vi "Create Runtime Configuration Files.vi"(6 "File Path":path=path "C:/dev/niveristand-runtime-configuration-example/Examples/Assets/Runtime Configuration - Subset.nivsruntimeconfig", 7 "Version":string="1.0", 8 "Error in":errorcluster, 9 "Creator":string="National Instruments", 10 "Description":string="Contains a sub set of channel information of Runtime Configuration Demo Custom Device which can be imported at runtime.", 11 "Name":string="TestRuntimeConfig") -> (0 "Error out":errorcluster)   [LabVIEW 2026]
uses:
  <vilib>/NI VeriStand/Custom Device API/Custom Device Channel Type.ctl
  <vilib>/NI/NI VeriStand Runtime Configuration File API/Runtime Configuration File API.lvlib
  <vilib>/NI VeriStand/Custom Device API/Custom Device API.lvlib
  Source/Runtime Configuration Support Example/Scripting/NIVS Runtime Configuration File Scripting API.lvlib
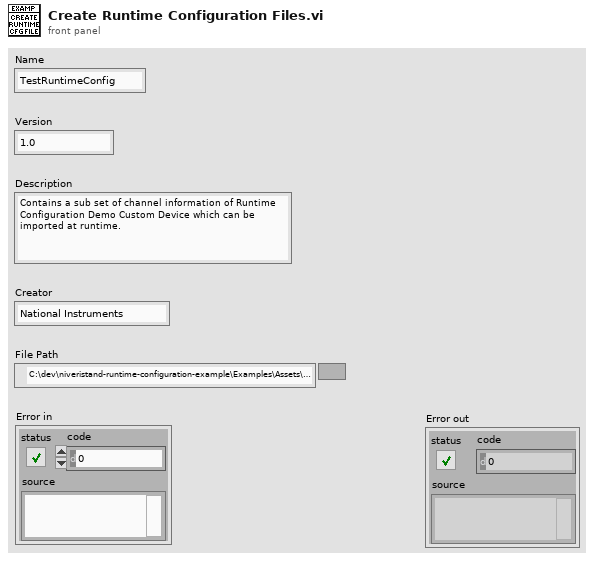
[diagram p1: front panel]
types:
  T1 = typedef "Custom Device API.lvlib/Custom Device Channel Type.ctl" = enum16{"Input", "Output"}
  T2 = typedef "Custom Device API.lvlib/Custom Device Item Ref.ctl" = u64
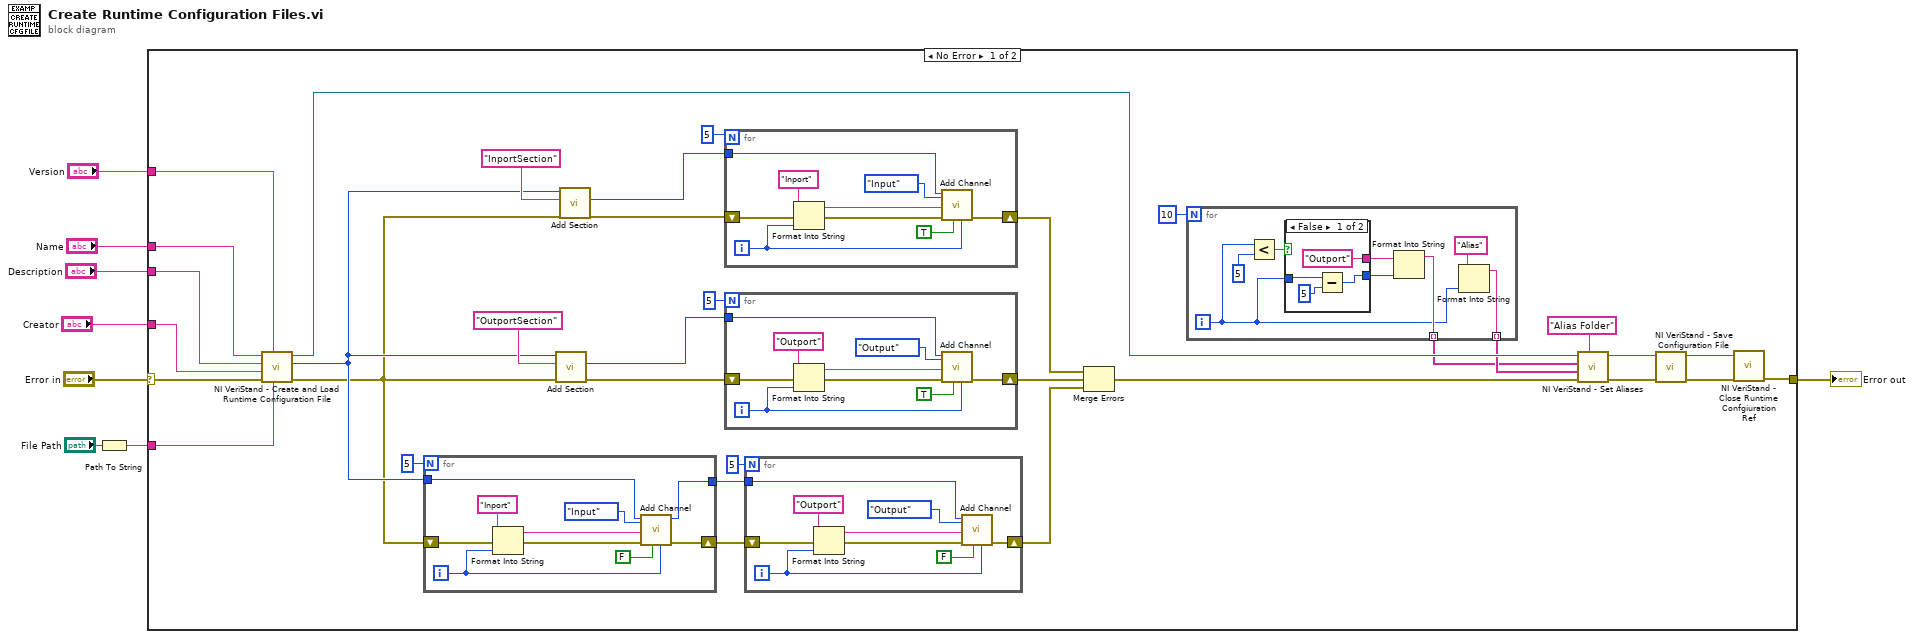
[diagram p0: block diagram]
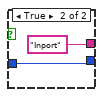
[diagram p2: hidden frame]
diagram:
  n1 = Path To String(path="File Path") -> (string=w1:string)
  n2 = case shown="No Error" "Error in" {
    selector: "Error in" -> [w41 w94]
    tunnel: [w10 w94] -> w8
    tunnel: "Name" -> [w37 _]
    tunnel: "Creator" -> [w36 _]
    tunnel: "Description" -> [w35 _]
    tunnel: "Version" -> [w34 _]
    tunnel: w1 -> [w33 _]
    frame No Error {
      n3 = call <vilib>:"NI VeriStand - Create and Load Runtime Configuration File.vi"("File Path"=w33, "Version"=w34, "Error in"=w41, "Creator"=w36, "Description"=w35, "Name"=w37) -> ("Error out"=w19:errorcluster, "Base Section ID"=w20:u64, "Runtime Configuration Ref"=w32:refnum<k24>)  [unwired: 3 in]
      n4 = for {
        N: 5 -> [_]
        shift-right: [w61] -> w18
        shift-left: w19 -> [w58]
        tunnel: w20 -> [w60]
        tunnel: [w59] -> w21
        i -> [w55]
        n5 = Format Into String(initial string="Inport", error in=w58, w55) -> (resulting string=w54:string, error out=w57:errorcluster)  [unwired: 1 in]
        n6 = call "Add Channel.vi"("SignalID"=w55, "Faultable"=FALSE, "error in"=w57, "Channel Type"=Custom_Device_Channel_Type."Input", "Channel Name"=w54, "Parent Ref in"=w60) -> ("error out"=w61:errorcluster, "Parent Ref out"=w59:T2)  [unwired: 3 in, 1 out]
      }
      n7 = call "Add Section.vi"("error in"=w19, "Section Name"="OutportSection", "Parent Ref in"=w20) -> ("error out"=w23:errorcluster, "Section Ptr"=w12:T2)  [unwired: 6 in, 1 out]
      n8 = call "Add Section.vi"("error in"=w19, "Section Name"="InportSection", "Parent Ref in"=w20) -> ("error out"=w40:errorcluster, "Section Ptr"=w13:T2)  [unwired: 6 in, 1 out]
      n9 = for {
        N: 5 -> [_]
        shift-right: [w93] -> w39
        shift-left: w40 -> [w91]
        tunnel: w13 -> [w92]
        i -> [w88]
        n10 = Format Into String(initial string="Inport", error in=w91, w88) -> (resulting string=w87:string, error out=w90:errorcluster)  [unwired: 1 in]
        n11 = call "Add Channel.vi"("SignalID"=w88, "Faultable"=TRUE, "error in"=w90, "Channel Type"=Custom_Device_Channel_Type."Input", "Channel Name"=w87, "Parent Ref in"=w92) -> ("error out"=w93:errorcluster)  [unwired: 3 in, 2 out]
      }
      n12 = for {
        N: 5 -> [_]
        shift-right: [w70] -> w22
        shift-left: w23 -> [w68]
        tunnel: w12 -> [w69]
        i -> [w65]
        n13 = Format Into String(initial string="Outport", error in=w68, w65) -> (resulting string=w64:string, error out=w67:errorcluster)  [unwired: 1 in]
        n14 = call "Add Channel.vi"("SignalID"=w65, "Faultable"=TRUE, "error in"=w67, "Channel Type"=Custom_Device_Channel_Type."Output", "Channel Name"=w64, "Parent Ref in"=w69) -> ("error out"=w70:errorcluster)  [unwired: 3 in, 2 out]
      }
      n15 = for {
        N: 5 -> [_]
        shift-right: [w51] -> w17
        shift-left: w18 -> [w49]
        tunnel: w21 -> [w50]
        i -> [w46]
        n16 = Format Into String(initial string="Outport", error in=w49, w46) -> (resulting string=w45:string, error out=w48:errorcluster)  [unwired: 1 in]
        n17 = call "Add Channel.vi"("SignalID"=w46, "Faultable"=FALSE, "error in"=w48, "Channel Type"=Custom_Device_Channel_Type."Output", "Channel Name"=w45, "Parent Ref in"=w50) -> ("error out"=w51:errorcluster)  [unwired: 3 in, 2 out]
      }
      n18 = Merge Errors(w39, w22, w17) -> (w38:errorcluster)
      n19 = for {
        N: 10 -> [_]
        tunnel: [w74] -> w24 mode=indexing
        tunnel: [w73] -> w25 mode=indexing
        i -> [w72]
        n20 = Less?(x=w72, y=5) -> (x < y?=w77:bool)
        n21 = case shown="False" w77 {
          tunnel: ["Outport" "Inport"] -> w78
          tunnel: w72 -> [w81 w84]
          tunnel: [w79 w84] -> w71
          frame False {
            n22 = Subtract(x=w81, y=5) -> (x-y=w79:i32)
          }
          frame True {
          }
        }
        n23 = Format Into String(initial string=w78, w71) -> (resulting string=w74:string)  [unwired: 2 in, 1 out]
        n24 = Format Into String(initial string="Alias", w72) -> (resulting string=w73:string)  [unwired: 2 in, 1 out]
      }
      n25 = call <vilib>:"NI VeriStand - Set Aliases.vi"("Runtime Alias Folder Name"="Alias Folder", "Error in"=w38, "Alias Names"=w25, "Referenced Channels"=w24, "Runtime Configuration Ref in"=w32) -> ("Error out"=w42:errorcluster, "Runtime Configuration Ref out"=w29:refnum<k24>)  [unwired: 4 in, 1 out]
      n26 = call <vilib>:"NI VeriStand - Save Configuration File.vi"("Error in"=w42, "Runtime Configuration Ref in"=w29) -> ("Error out"=w11:errorcluster, "Runtime Configuration Ref out"=w9:refnum<k24>)  [unwired: 7 in, 1 out]
      n27 = call <vilib>:"NI VeriStand - Close Runtime Confgiuration Ref.vi"("error in"=w11, "Runtime Configuration Ref in"=w9) -> ("error out"=w10:errorcluster)  [unwired: 9 in]
    }
    frame Error {
    }
  }
  "Error out" <- w8
